vi "ProgramBitstreamWriteMeasurementFile.vi"() -> ()   [LabVIEW 2009]
panel:
  in  "Results File":path
  in  "Bitstream Filenames File":path
  out "return code":i32
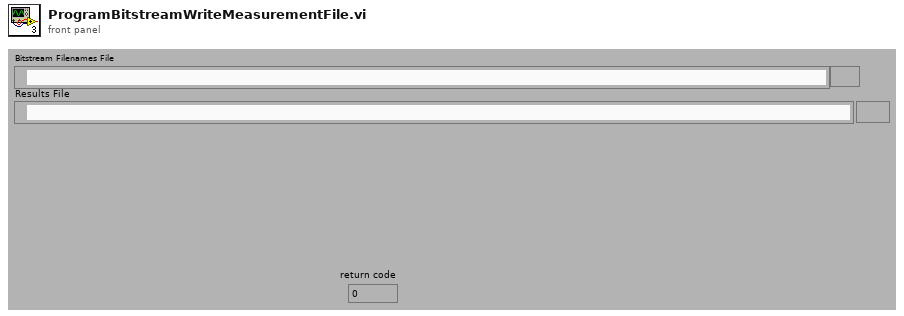
[diagram p1: front panel]
types:
  T1 = enum16{"open", "replace", "create", "open or create", "replace or create", "replace or create with confirmation"}
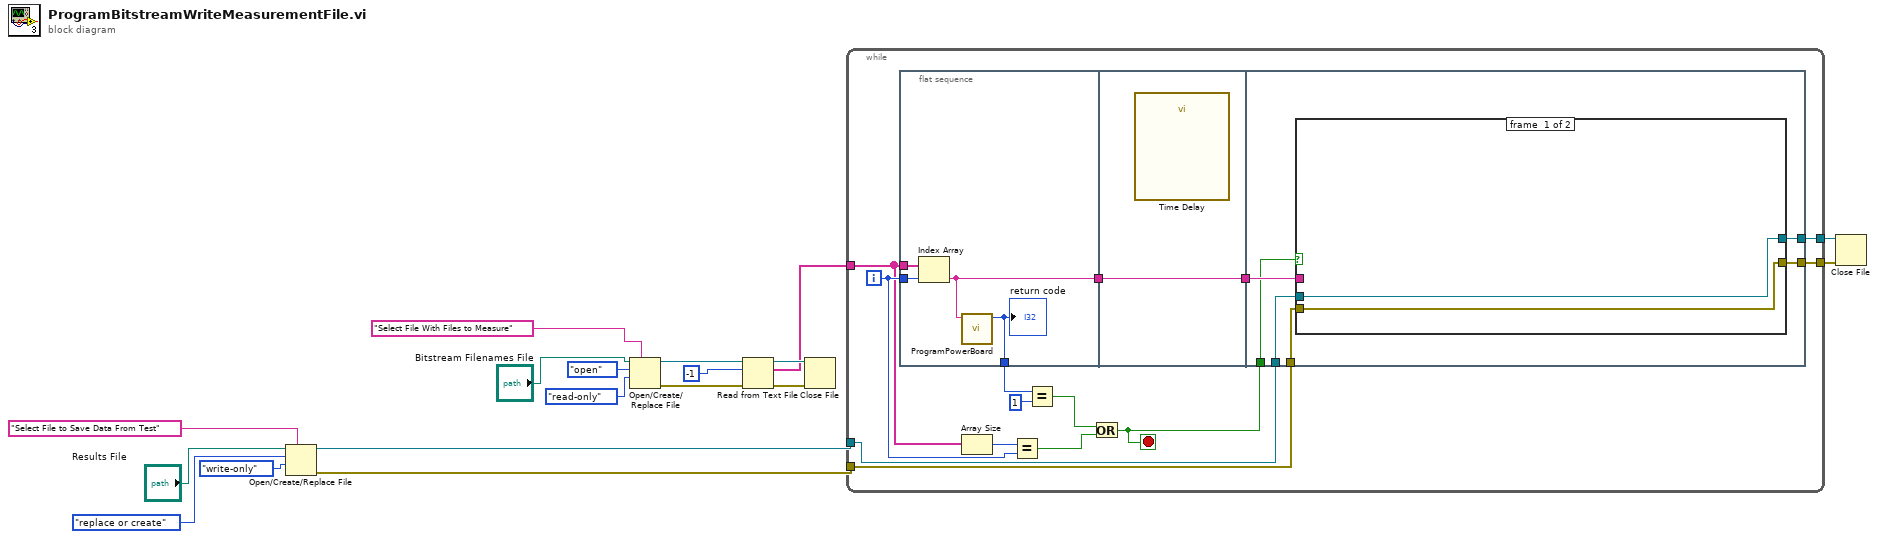
[diagram p0: block diagram]
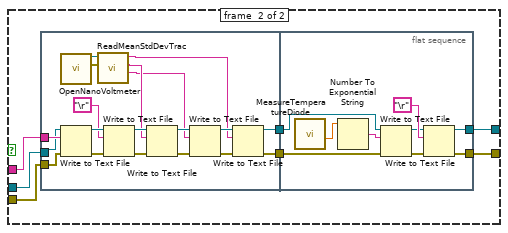
[diagram p2: hidden frame]
diagram:
  n1 = Open/Create/Replace File(file path (use dialog)="Results File", prompt="Select File to Save Data From Test", operation (0:open)=T1."replace or create", access (0:read/write)=enum16{"read/write", "read-only", "write-only"}."write-only") -> (refnum out=w14:refnum<file>, error out=w11:errorcluster)  [unwired: 2 in, 1 out]
  n2 = Open/Create/Replace File(file path (use dialog)="Bitstream Filenames File", prompt="Select File With Files to Measure", operation (0:open)=T1."open", access (0:read/write)=enum16{"read/write", "read-only", "write-only"}."read-only") -> (refnum out=w6:refnum<file>, error out=w3:errorcluster)  [unwired: 2 in, 1 out]
  n3 = Read from Text File(file (use dialog)=w6, count=-1, error in=w3) -> (refnum out=w5:refnum<file>, text=w1:string[], error out=w4:errorcluster)  [unwired: 1 in, 1 out]
  n4 = Close File(refnum=w5, error in=w4) -> ()  [unwired: 2 out]
  n5 = while {
    tunnel: w1 -> [w27]
    tunnel: w14 -> [w25]
    tunnel: [w24] -> w13
    tunnel: [w23] -> w12
    tunnel: w11 -> [w22]
    i -> [w28]
    stop <- w19 stop-if-true
    n6 = flat-sequence {
      tunnel: [w36] -> w31
      tunnel: w27 -> [w34]
      tunnel: w28 -> [w35]
      tunnel: [w33] -> w21
      tunnel: w21 -> [w37]
      tunnel: [w37] -> w20
      tunnel: w20 -> [w39]
      tunnel: w25 -> [w41]
      tunnel: [w43] -> w24
      tunnel: [w42] -> w23
      tunnel: w22 -> [w40]
      tunnel: w19 -> [w38]
      frame #0 {
        n7 = Index Array(array=w34, index=w35) -> (element=w33:string)
        n8 = call "ProgramPowerBoard.vi"("BitstreamFilename"=w33) -> ("return code"=w36:i32)  [unwired: 10 in]
        "return code" <- w36
      }
      frame #1 {
        n9 = call "Time Delay"() -> ()  [unwired: 11 in, 1 out]
      }
      frame #2 {
        n10 = case shown="True" w38 {
          tunnel: [w44 w47] -> w43
          tunnel: [w45 w46] -> w42
          tunnel: w41 -> [w44 w51]
          tunnel: w40 -> [w45 w50]
          tunnel: w39 -> [_ w52]
          frame #0 {
          }
          frame #1 {
            n11 = flat-sequence {
              tunnel: w52 -> [w62]
              tunnel: w51 -> [w61]
              tunnel: w50 -> [w60]
              tunnel: [w59] -> w49
              tunnel: [w58] -> w48
              tunnel: w49 -> [w74]
              tunnel: w48 -> [w75]
              tunnel: [w73] -> w47
              tunnel: [w72] -> w46
              frame #0 {
                n12 = call "OpenNanoVoltmeter.vi"() -> ("error out"=w53:errorcluster, "reference out"=w54:refnum<visa-resource-name>)  [unwired: 8 in]
                n13 = Write to Text File(file (use dialog)=w61, text=w62, error in=w60) -> (refnum out=w64:refnum<file>, error out=w65:errorcluster)  [unwired: 1 in, 1 out]
                n14 = call "ReadMeanStdDevTrac.vi"("error in"=w53, "reference in 3"=w54) -> ("STDDEV"=w55:string, "MEAN"=w56:string, "TRACEr"=w57:string)  [unwired: 5 in, 2 out]
                n15 = Write to Text File(file (use dialog)=w64, text="\r", error in=w65) -> (refnum out=w71:refnum<file>, error out=w66:errorcluster)  [unwired: 1 in, 1 out]
                n16 = Write to Text File(file (use dialog)=w71, text=w56, error in=w66) -> (refnum out=w70:refnum<file>, error out=w67:errorcluster)  [unwired: 1 in, 1 out]
                n17 = Write to Text File(file (use dialog)=w70, text=w55, error in=w67) -> (refnum out=w69:refnum<file>, error out=w68:errorcluster)  [unwired: 1 in, 1 out]
                n18 = Write to Text File(file (use dialog)=w69, text=w57, error in=w68) -> (refnum out=w59:refnum<file>, error out=w58:errorcluster)  [unwired: 1 in, 1 out]
              }
              frame #1 {
                n19 = call "MeasureTemperatureDiode.vi"() -> ("Celcius"=w80:dbl)  [unwired: 8 in, 3 out]
                n20 = Number To Exponential String(number=w80) -> (E-format string=w79:string)  [unwired: 3 in]
                n21 = Write to Text File(file (use dialog)=w74, text=w79, error in=w75) -> (refnum out=w77:refnum<file>, error out=w76:errorcluster)  [unwired: 1 in, 1 out]
                n22 = Write to Text File(file (use dialog)=w77, text="\r", error in=w76) -> (refnum out=w73:refnum<file>, error out=w72:errorcluster)  [unwired: 1 in, 1 out]
              }
            }
          }
        }
      }
    }
    n23 = Array Size(array=w27) -> (size(s)=w26:i32)
    n24 = Equal?(x=w26, y=w28) -> (x = y?=w32:bool)
    n25 = Equal?(x=w31, y=1) -> (x = y?=w29:bool)
    n26 = Or(x=w29, y=w32) -> (x .or. y?=w19:bool)
  }
  n27 = Close File(refnum=w13, error in=w12) -> ()  [unwired: 2 out]
